vi "Read Digital Port.vi"(8 "error in (no error)":errorcluster, 11 "DIO in":refnum<class "DIO.lvclass">) -> (0 "error out":errorcluster, 2 "Boolean":bool, 3 "DIO out":refnum<class "DIO.lvclass">)   [LabVIEW 2021, in "HAL.lvlib" / "DIO.lvclass"]
uses:
  DIO.lvclass
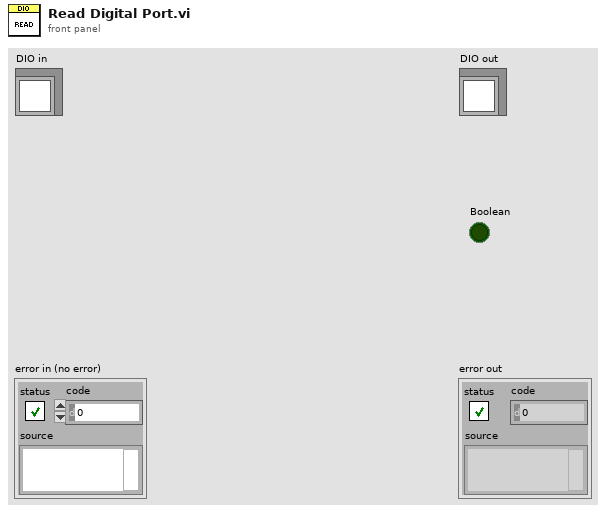
[diagram p1: front panel]
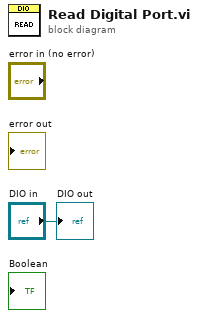
[diagram p0: block diagram]
diagram:
  "DIO out" <- "DIO in"
